vi "DAQmx Read (Digital Bool 1Line 1Point).vi"(0 "task/channels in":refnum<k21>, 9 "timeout":dbl=10.0 format="%0.2f", 11 "error in":errorcluster) -> (4 "task out":refnum<k21>, 6 "data":bool, 15 "error out":errorcluster)   [LabVIEW 2022 SP3]
doc: "Reads a single Boolean sample from a task that contains a digital input channel composed of a single line."
uses:
  nilvaiu.dll
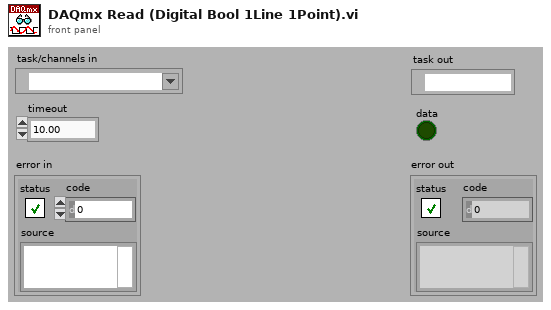
[diagram p1: front panel]
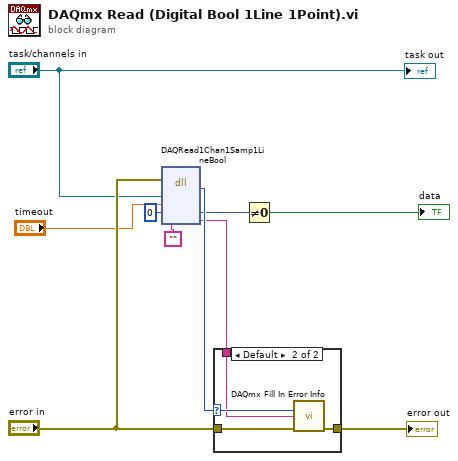
[diagram p0: block diagram]
diagram:
  n1 = dll-call lib="nilvaiu.*" fn="DAQRead1Chan1Samp1LineBool"(error in="error in", "taskID"="task/channels in", "timeout"="timeout", "data"=u8 0, "extendedErrorInfo"="") -> (w5:i32, "data"=w2:u8, "extendedErrorInfo"=w3:string)  [unwired: 3 in, 3 out]
  n2 = case shown="Default" w5 {
    selector: w5 -> [_ w14]
    tunnel: "error in" -> [w11 w15]
    tunnel: [w11 w13] -> w9
    tunnel: w3 -> [_ w12]
    frame 0 {
    }
    frame Default {
      n3 = call "DAQmx Fill In Error Info.vi"("status code"=w14, "extended error info"=w12, "error in"=w15) -> ("error out"=w13:errorcluster)  [unwired: 1 in, 11 out]
    }
  }
  "error out" <- w9
  n4 = Not Equal To 0?(x=w2) -> (x != 0?=→"data":bool)
  "task out" <- "task/channels in"
